vi "Plugin ID to Tree Items.vi"(8 "error in (no error)":errorcluster, 9 "Plugin ID":string, 10 "Indent":i32, 11 "Application Data in":T2) -> (0 "error out":errorcluster, 2 "tree items":T1(array[cluster]), 3 "Application Data out":T2)   [LabVIEW 2017]
uses:
  Application Data.ctl
  DSF Configuration API/1.0.0/Public/Controls/DSF Config Data RefNum.ctl
  Window State.ctl
  Tree Item Type.ctl
  DSF Configuration API/1.0.0/Public/Read Item/Read Plugin.vi
  DSF Configuration API/1.0.0/Public/Read Item/Read Settings.vi
  DSF Configuration API/1.0.0/DSF Configuration API.lvlib
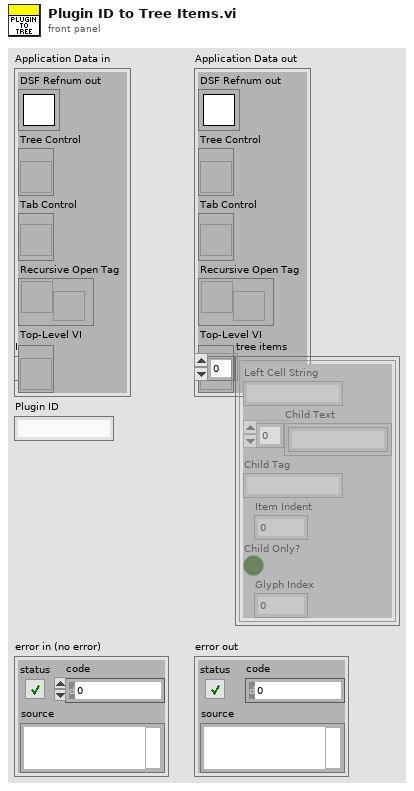
[diagram p1: front panel]
types:
  T1 = cluster{"Left Cell String":string, "Child Text":string[], "Child Tag":string, "Item Indent":i32, "Child Only?":bool, "Glyph Index":i32}[]
  T2 = typedef "Application Data.ctl" = cluster{"DSF Refnum out":T3, "Tree Control":refnum<vi>, "Tab Control":refnum<vi>, "Recursive Open Tag":refnum<user-event>, "Top-Level VI":refnum<vi>}
  T3 = typedef "DSF Configuration API.lvlib/DSF Config Data RefNum.ctl" = refnum<k1>
  T4 = typedef "Tree Item Type.ctl" = enum16{"Plugin", "Group", "Transfer", "Channel", "Setting"}
  T5 = typedef "DSF Configuration API.lvlib/DSF Plugin Info.ctl" = cluster{"type":string, "timing":T6, "group ids":string[], "settings id":string}
  T6 = typedef "DSF Configuration API.lvlib/DSF Timing Info.ctl" = cluster{"decimation":i32, "offset":i32}
  T7 = cluster{"Left Cell String":string, "Child Text":string[], "Child Tag":string, "Item Indent":i32, "Child Only?":bool, "Glyph Index":i32}
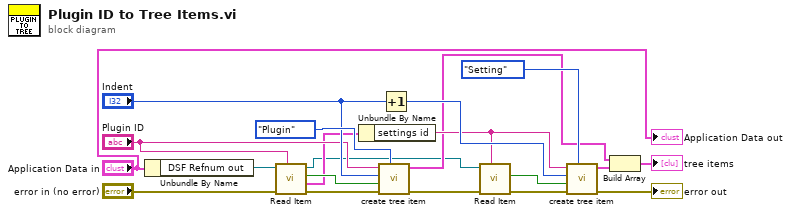
[diagram p0: block diagram]
diagram:
  n1 = Unbundle By Name("Application Data in") -> ("DSF Refnum out"=w3:T3)
  n2 = call-poly "Read Item.vi"("name"="Plugin ID", "error in (no error)"="error in (no error)", "refnum"=w3) -> ("error out"=w9:errorcluster, "value"=w11:T5, "found?"=w12:bool, "refnum out"=w2:T3)  [unwired: 5 in]
  n3 = Unbundle By Name(w11) -> ("settings id"=w14:string)
  n4 = call "create tree item.vi"("Item Type"=Tree_Item_Type."Plugin", "error in"=w9, "found?"=w12, "Indent"="Indent", "Left Cell String"="Plugin ID") -> ("error out"=w8:errorcluster, "Item"=w6:T7)  [unwired: 5 in]
  n5 = Increment(x="Indent") -> (x+1=w17:i32)
  n6 = call-poly "Read Item.vi"("name"=w14, "error in (no error)"=w8, "refnum"=w2) -> ("error out"=w18:errorcluster, "found?"=w16:bool)  [unwired: 5 in, 2 out]
  n7 = call "create tree item.vi"("Item Type"=Tree_Item_Type."Setting", "error in"=w18, "found?"=w16, "Indent"=w17, "Left Cell String"=w14) -> ("error out"=→"error out":errorcluster, "Item"=w5:T7)  [unwired: 5 in]
  n8 = Build Array(w6, w5) -> (→"tree items":T1)
  "Application Data out" <- "Application Data in"
